vi "Asylum_Driver_LithographyObjects.vi"(5 "Writing Setpoint":dbl=0.1 format="%#_13g", 6 "Interpolation":dbl format="%#_13g", 7 "Move Setpoint":dbl=-1.3 format="%#_13g", 8 "error in (no error)":errorcluster, 9 "Offsets":cluster{"X":dbl, "Y":dbl}, 10 "Lithography Data":T2(array[cluster]), 11 "Application":refnum<k7>) -> (0 "error out":errorcluster)   [LabVIEW 2020]
uses:
  <userlib>/LevyLab/Relay Box/Type_defs/Resistor--enum.ctl
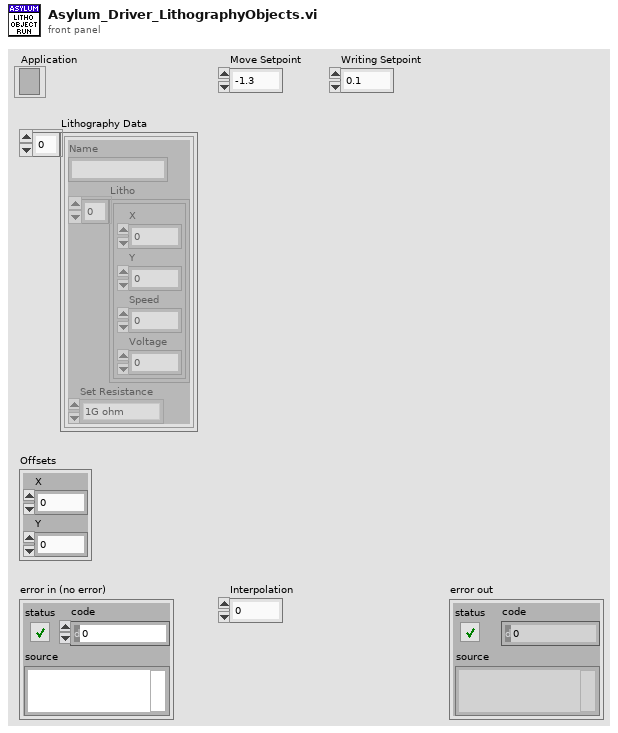
[diagram p1: front panel]
types:
  T1 = typedef "Resistor--enum.ctl" = enum16{"open", "discharge tip", "0 ohms", "100k ohm", "10M ohm", "1G ohm"}
  T2 = cluster{"Name":string, "Litho":cluster{"X":dbl, "Y":dbl, "Speed":dbl, "Voltage":dbl}[], "Set Resistance":T1}[]
  T3 = cluster{"X":dbl, "Y":dbl, "Speed":dbl, "Voltage":dbl}[]
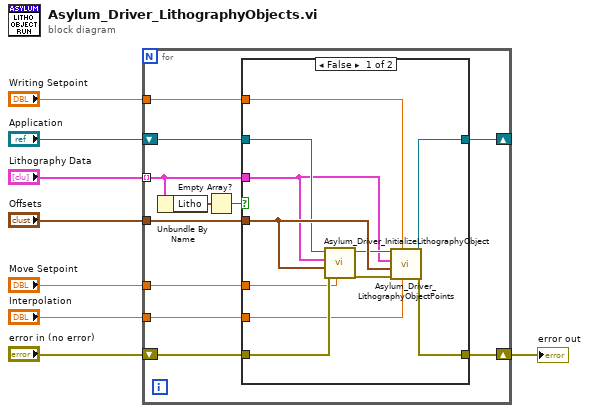
[diagram p0: block diagram]
diagram:
  n1 = for {
    tunnel: "Lithography Data" -> [w13] mode=indexing
    tunnel: "Offsets" -> [w16]
    shift-right: [w18] -> w7
    shift-left: "error in (no error)" -> [w19]
    tunnel: "Interpolation" -> [w17]
    tunnel: "Move Setpoint" -> [w11]
    tunnel: "Writing Setpoint" -> [w10]
    shift-right: [w9] -> _
    shift-left: "Application" -> [w15]
    n2 = Unbundle By Name(w13) -> ("Litho"=w12:T3)
    n3 = Empty Array?(array=w12) -> (empty?=w14:bool)
    n4 = case shown="False" w14 {
      tunnel: w19 -> [w28 w32]
      tunnel: w17 -> [w27 _]
      tunnel: [w29 w32] -> w18
      tunnel: w13 -> [w23 _]
      tunnel: w16 -> [w26 _]
      tunnel: w15 -> [w25 w31]
      tunnel: w11 -> [w21 _]
      tunnel: w10 -> [w22 _]
      tunnel: [w20 w31] -> w9
      frame False {
        n5 = call "Asylum_Driver_InitializeLithographyObject.vi"("Z Setpoint"=w21, "error in (no error)"=w28, "Offsets"=w26, "Pattern Data"=w23, "Application"=w25) -> ("error out"=w30:errorcluster, "Application"=w24:refnum<k7>)  [unwired: 5 in]
        n6 = call "Asylum_Driver_LithographyObjectPoints.vi"("Interpolation"=w27, "Writing Setpoint"=w22, "error in (no error)"=w30, "Offsets"=w26, "Pattern Data"=w23, "Application"=w24) -> ("error out"=w29:errorcluster, "Application"=w20:refnum<k7>)  [unwired: 4 in]
      }
      frame True {
      }
    }
  }
  "error out" <- w7
